vi "convertCompassRawDataToDeg.vi"(0 "raw x":sgl, 7 "raw y":sgl, 11 "raw z":sgl) -> (4 "x":sgl, 8 "y":sgl, 14 "deg":sgl, 15 "z":sgl)   [LabVIEW 2023]
panel:
  in  "z scale [µT]":sgl=2500.0 format="%#_13g"
  in  "x,y scale [µT]":sgl=1300.0 format="%#_13g"
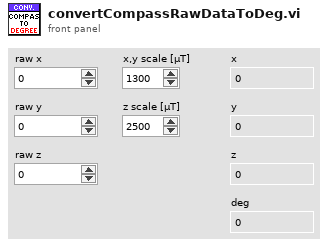
[diagram p1: front panel]
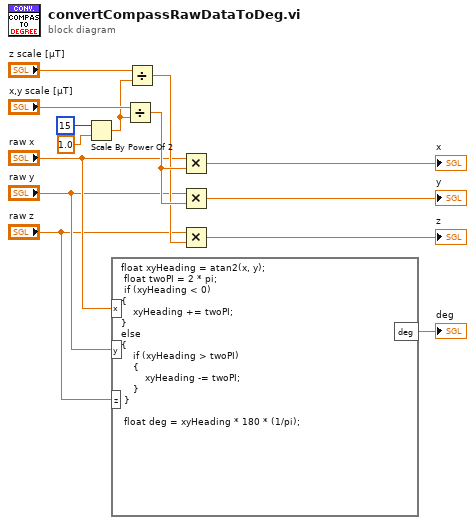
[diagram p0: block diagram]
diagram:
  n1 = Scale By Power Of 2(n=i16 15, x=sgl 1.0) -> (x*2^n=w6:sgl)
  n2 = formula code="float xyHeading = atan2(x, y);\n\tfloat twoPI = 2 * pi;\n\tif (xyHeading < 0)\n{\n    xyHeading += twoPI;\n}\nelse \n{\n    if (xyHeading > twoPI) \n    { \n        xyHeading -= twoPI;\n    }\n\t}\n\t\n\tfloat deg = xyHeading * 180 * (1/pi);"("x"="raw x", "y"="raw y", "z"="raw z") -> ("deg"=→"deg":dbl)
  n3 = Divide(x="x,y scale [µT]", y=w6) -> (x/y=w8:sgl)
  n4 = Divide(x="z scale [µT]", y=w6) -> (x/y=w5:sgl)
  n5 = Multiply(x="raw x", y=w8) -> (x*y=→"x":sgl)
  n6 = Multiply(x="raw y", y=w8) -> (x*y=→"y":sgl)
  n7 = Multiply(x="raw z", y=w5) -> (x*y=→"z":sgl)
